vi "readTag.vi"(8 "error in (no error)":errorcluster, 11 "cRIO in":refnum<class "cRIO.lvclass">) -> (0 "error out":errorcluster, 3 "cRIO out":refnum<class "cRIO.lvclass">)   [LabVIEW 2020, in "cRIO.lvclass"]
uses:
  cRIO.lvclass
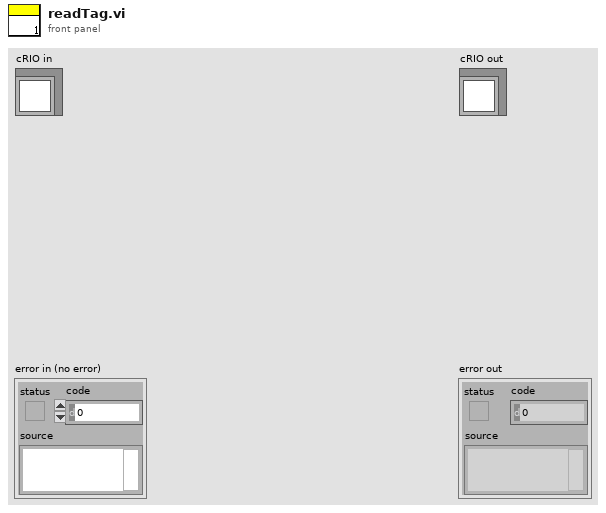
[diagram p1: front panel]
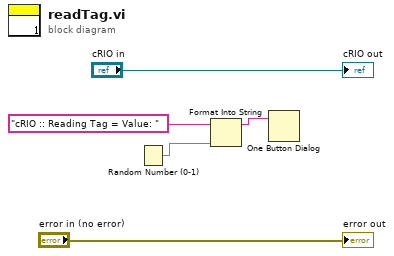
[diagram p0: block diagram]
diagram:
  n1 = Random Number (0-1)() -> (number: 0 to 1=w2:dbl)
  n2 = Format Into String(initial string="cRIO :: Reading Tag = Value: " ("message"), w2) -> (resulting string=w1:string)  [unwired: 2 in, 1 out]
  n3 = One Button Dialog(message=w1) -> ()  [unwired: 1 in, 1 out]
  "error out" <- "error in (no error)"
  "cRIO out" <- "cRIO in"
